vi "Configure Filter.vi"(8 "error in (no error)":errorcluster, 10 "Current Filter Settings":T1={"Level Filter"={"Warning"=FALSE, "Debug"=FALSE, "Info"=FALSE, "Error"=FALSE, "Critical"=FALSE}, "Source Filter"={"Source"="", "Exclude Match?"=TRUE, "Exact Match?"=TRUE}, "Keyword Filter"={"Keywords"=[], "Exclude Match?"=TRUE}}, 11 "ConsoleView Sink in":refnum<class "ConsoleView.lvclass">) -> (0 "error out":errorcluster, 3 "ConsoleView Sink out":refnum<class "ConsoleView.lvclass">)   [LabVIEW 2020, in "MVA Framework.lvlib" / "ConsoleView.lvlib" / "ConsoleView.lvclass"]
uses:
  ConsoleView.lvclass
  TypeDef/FilterConfig.ctl
  Composed Log/ILogFilter/ILogFilter.lvclass
  ConsoleView.lvclass/ConsoleView.ctl
  Filters/Event Keyword Filter/Event Keyword Filter.lvclass
  Filters/Event Source Filter/Event Source Filter.lvclass
  Filters/Event Level Filter/Event Level Filter.lvclass
  Filters/Compound Filter/Compound Filter.lvclass
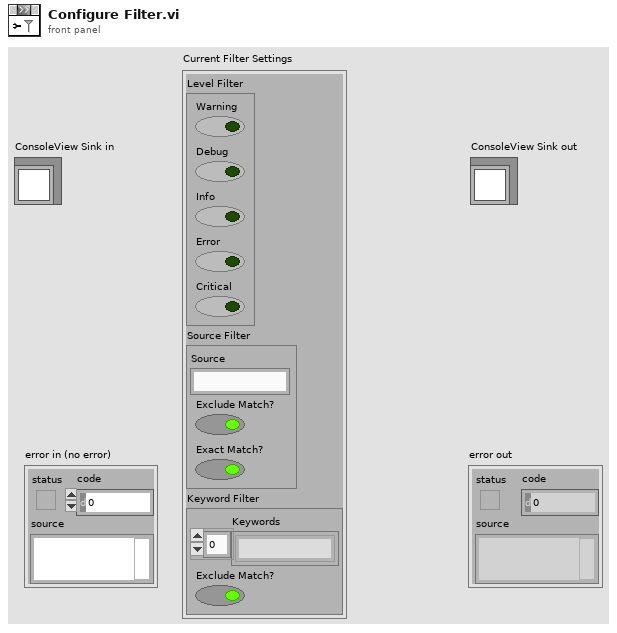
[diagram p1: front panel]
types:
  T1 = typedef "MVA Framework.lvlib/ConsoleView.lvlib/ConsoleView.lvclass/FilterConfig.ctl" = cluster{"Level Filter":cluster{"Warning":bool, "Debug":bool, "Info":bool, "Error":bool, "Critical":bool}, "Source Filter":cluster{"Source":string, "Exclude Match?":bool, "Exact Match?":bool}, "Keyword Filter":cluster{"Keywords":string[], "Exclude Match?":bool}}
  T2 = cluster{"Debug":bool, "Info":bool, "Warning":bool, "Error":bool, "Critical":bool}
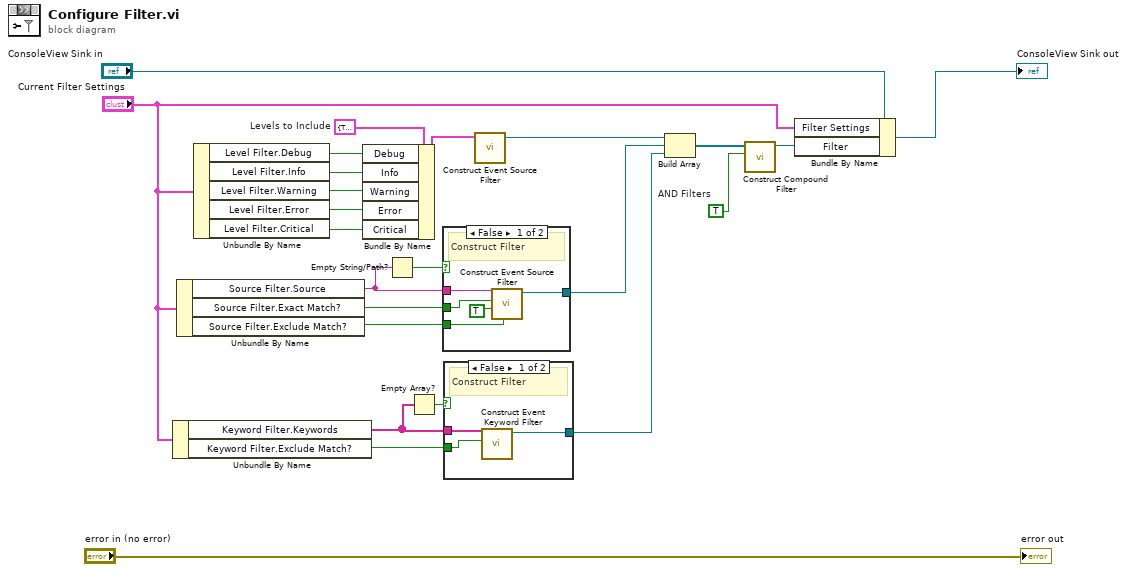
[diagram p0: block diagram]
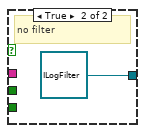
[diagram p2: hidden frame]
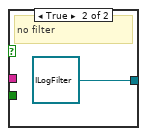
[diagram p3: hidden frame]
diagram:
  w7 = T2 {"Debug"=TRUE, "Info"=TRUE, "Warning"=TRUE, "Error"=TRUE, "Critical"=TRUE}  # Levels to Include
  w19 = TRUE  # AND Filters
  n1 = Unbundle By Name("Current Filter Settings") -> ("Keyword Filter.Keywords"=w13:string[], "Keyword Filter.Exclude Match?"=w12:bool)
  n2 = Unbundle By Name("Current Filter Settings") -> ("Source Filter.Source"=w10:string, "Source Filter.Exact Match?"=w9:bool, "Source Filter.Exclude Match?"=w8:bool)
  n3 = Unbundle By Name("Current Filter Settings") -> ("Level Filter.Debug"=w5:bool, "Level Filter.Info"=w1:bool, "Level Filter.Warning"=w2:bool, "Level Filter.Error"=w3:bool, "Level Filter.Critical"=w4:bool)
  n4 = Bundle By Name(cluster=w7, "Debug"=w5, "Info"=w1, "Warning"=w2, "Error"=w3, "Critical"=w4) -> (w6:T2)
  n5 = Empty String/Path?(string/path=w10) -> (empty?=w11:bool)
  n6 = Empty Array?(array=w13) -> (empty?=w14:bool)
  n7 = case shown="False" w11 {
    tunnel: [w28 refnum<class "ILogFilter.lvclass"> refnum ("Composed Log.lvlib:ILogFilter.lvclass")] -> w22
    tunnel: w10 -> [w27 _]
    tunnel: w9 -> [w26 _]
    tunnel: w8 -> [w25 _]
    frame False {
      # "Construct Filter"
      n8 = call "Construct Event Source Filter.vi"("Exclude?(F)"=w25, "Ignore Case?"=TRUE, "Exact Match?"=w26, "Source ID"=w27) -> ("Compound Filter out"=w28:refnum<class "Event Source Filter.lvclass">)  [unwired: 6 in, 1 out]
    }
    frame True {
      # "no filter"
    }
  }
  n9 = case shown="False" w14 {
    tunnel: [w33 refnum<class "ILogFilter.lvclass"> refnum ("Composed Log.lvlib:ILogFilter.lvclass")] -> w21
    tunnel: w13 -> [w32 _]
    tunnel: w12 -> [w31 _]
    frame False {
      # "Construct Filter"
      n10 = call "Construct Event Keyword Filter.vi"("Exclude Matches?"=w31, "Keywords"=w32) -> ("Event Keyword Filter out"=w33:refnum<class "Event Keyword Filter.lvclass">)  [unwired: 9 in]
    }
    frame True {
      # "no filter"
    }
  }
  n11 = call "Construct Event Source Filter.vi"("Levels to Include (All)"=w6) -> ("Event Level Filter out"=w23:refnum<class "Event Level Filter.lvclass">)  [unwired: 10 in]
  n12 = Build Array(w23, w22, w21) -> (w20:refnum<class "ILogFilter.lvclass">[])
  n13 = call "Construct Compound Filter.vi"("AND Filters? (Default T, F OR)"=w19, "Filters"=w20) -> ("Compound Filter out"=w16:refnum<class "Compound Filter.lvclass">)  [unwired: 8 in, 1 out]
  n14 = Bundle By Name(cluster="ConsoleView Sink in", "Filter Settings"="Current Filter Settings", "Filter"=w16) -> (→"ConsoleView Sink out":refnum<class "ConsoleView.lvclass">)
  "error out" <- "error in (no error)"
